vi "Pause.vi"(8 "error in (no error)":errorcluster, 11 "VICI Settings In":T1) -> (0 "error out":errorcluster, 1 "Connection Error":bool, 3 "VICI Settings Out":T1)   [LabVIEW 2018, in "VICI M6 M50 Party Mode.lvlib"]
uses:
  VICI M6 M50 Party Mode.lvlib
  Settings Cluster.ctl
  VICI Global Library.lvlib
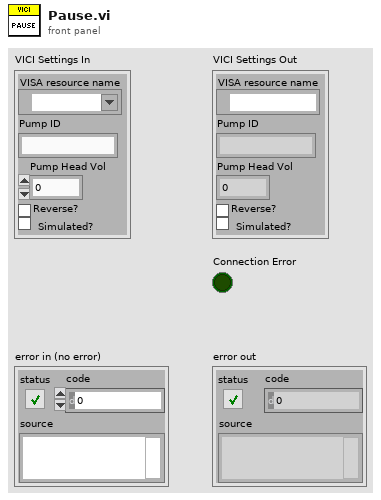
[diagram p1: front panel]
types:
  T1 = typedef "VICI M6 M50 Party Mode.lvlib/Settings Cluster.ctl" = cluster{"VISA resource name":refnum<visa-resource-name>, "Pump ID":string, "Pump Head Vol":dbl, "Reverse?":bool, "Simulated?":bool}
  T2 = typedef "VICI M6 M50 Party Mode.lvlib/VICI Global Library.lvlib/VICI Global.ctl" = cluster{"Busy":bool, "VISA #":string, "Current Pump":string, "Current Function":string, "Pump Array":string[], "Last Success":timestamp, "ID Queue":string[]}
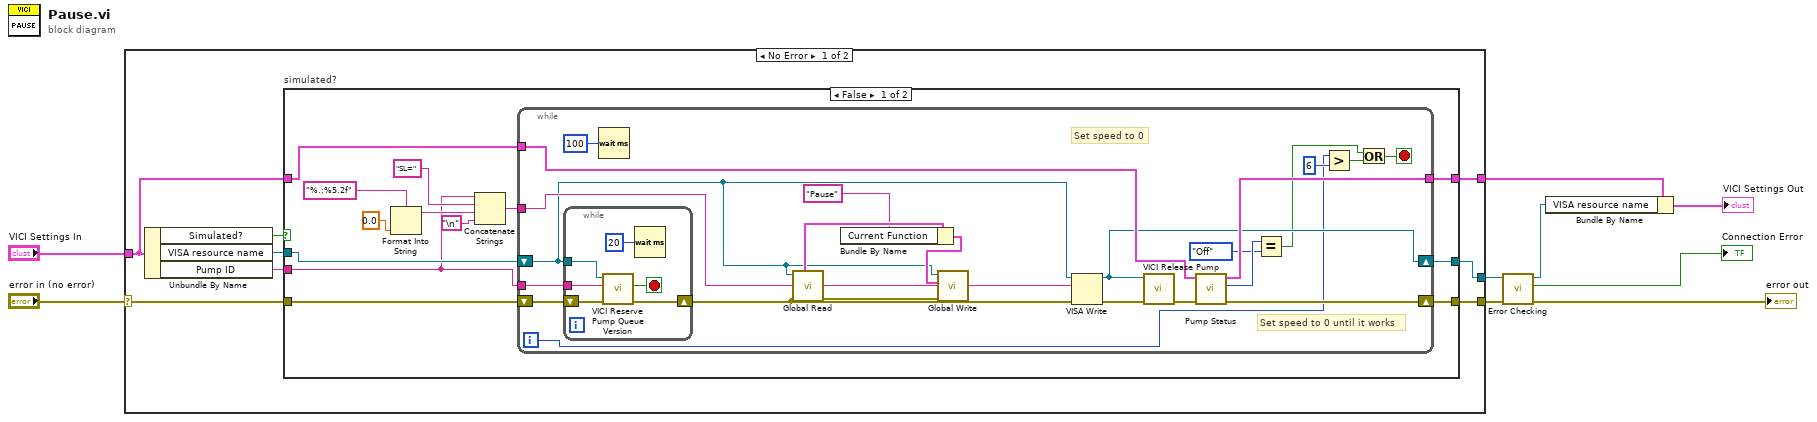
[diagram p0: block diagram]
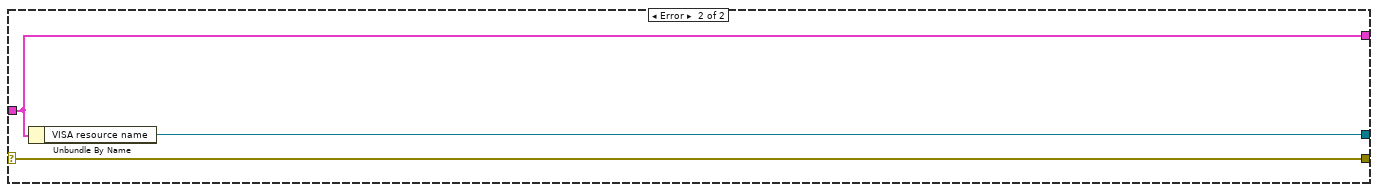
[diagram p3: hidden frame]
diagram:
  n1 = case shown="No Error" "error in (no error)" {
    selector: "error in (no error)" -> [w17 w65]
    tunnel: [w13 w64] -> w3
    tunnel: "VICI Settings In" -> [w14 w64]
    tunnel: [w16 w63] -> w7
    tunnel: [w15 w65] -> w6
    frame No Error {
      n2 = Unbundle By Name(w14) -> ("Simulated?"=w11:bool, "VISA resource name"=w12:refnum<visa-resource-name>, "Pump ID"=w10:string)
      n3 = case "simulated?" shown="False" w11 {
        tunnel: [w28 w62] -> w16
        tunnel: w12 -> [w30 w62]
        tunnel: w17 -> [w29 w61]
        tunnel: [w27 w61] -> w15
        tunnel: w14 -> [w26 w60]
        tunnel: [w25 w60] -> w13
        tunnel: w10 -> [w18 _]
        frame False {
          n4 = Format Into String(format string="%.;%5.2f", 0.0 ("input 1")) -> (resulting string=w24:string)  [unwired: 2 in, 1 out]
          n5 = Concatenate Strings(w18, "SL=" ("string"), w24, "\n") -> (w19:string)
          n6 = while {
            shift-right: [w42] -> w28
            shift-left: w30 -> [w32]
            shift-right: [w53] -> w27
            shift-left: w29 -> [w45]
            tunnel: w26 -> [w52]
            tunnel: [w51] -> w25
            tunnel: w19 -> [w47]
            tunnel: w18 -> [w46]
            i -> [w37]
            stop <- w38 stop-if-true
            # "Set speed to 0 until it works"
            # "Set speed to 0"
            n7 = while {
              tunnel: w32 -> [w58]
              tunnel: w46 -> [w57]
              shift-right: [w54] -> w31
              shift-left: w45 -> [w56]
              stop <- w55 stop-if-true
              n8 = call "VICI Reserve Pump Queue Version.vi"("error in (no error)"=w56, "Pump ID"=w57, "VISA # in"=w58) -> ("error out"=w54:errorcluster, "Loop Completed"=w55:bool)  [unwired: 6 in, 1 out]
              n9 = Wait (ms)(milliseconds to wait=u32 20) -> ()  [unwired: 1 out]
            }
            n10 = Wait (ms)(milliseconds to wait=u32 100) -> ()  [unwired: 1 out]
            n11 = call "Global Read.vi"("VISA #"=w32, "error in (no error)"=w31) -> ("Global for this VISA"=w35:T2, "error out"=w36:errorcluster)  [unwired: 2 in, 5 out]
            n12 = Bundle By Name(cluster=w35, "Current Function"="Pause") -> (w34:T2)
            n13 = call "Global Write.vi"("error in (no error)"=w36, "VICI Global"=w34, "VISA # in"=w32) -> ()  [unwired: 7 in, 2 out]
            n14 = VISA Write(VISA resource name=w32, write buffer=w47, error in (no error)=w31) -> (VISA resource name out=w42:refnum<visa-resource-name>, error out=w44:errorcluster)  [unwired: 1 out]
            n15 = call "VICI Release Pump.vi"("error in (no error)"=w44, "VISA # in"=w42) -> ("error out"=w43:errorcluster)  [unwired: 8 in, 1 out]
            n16 = call "Pump Status.vi"("error in (no error)"=w43, "VICI Settings In"=w52) -> ("error out"=w53:errorcluster, "Pump On?"=w49:enum16{"Off", "On", "Not Initialized"}, "VICI Settings Out"=w51:T1)  [unwired: 6 in, 1 out]
            n17 = Equal?(x=w49, y=enum16{"Off", "On", "Not Initialized"}."Off") -> (x = y?=w39:bool)
            n18 = Greater?(x=w37, y=6) -> (0:w40:bool)
            n19 = Or(x=w39, y=w40) -> (x .or. y?=w38:bool)
          }
        }
        frame True {
        }
      }
    }
    frame Error {
      n20 = Unbundle By Name(w64) -> ("VISA resource name"=w63:refnum<visa-resource-name>)
    }
  }
  n21 = call "Error Checking.vi"("error in (no error)"=w6, "VISA resource name"=w7) -> ("error out"=→"error out":errorcluster, "Connection Error"=→"Connection Error":bool, "VISA resource name"=w4:refnum<visa-resource-name>)  [unwired: 7 in]
  n22 = Bundle By Name(cluster=w3, "VISA resource name"=w4) -> (→"VICI Settings Out":T1)
